vi "ReadINIfile.vi"(6 "Delete INI File First? (F)":bool, 8 "error in (no error)":errorcluster) -> (0 "error out":errorcluster, 2 "Existing Addresses":string[][](array[string]), 3 "refnum out":T1)   [LabVIEW 2009]
uses:
  <vilib>/Utility/config.llb/Config Data RefNum.ctl
  <vilib>/Utility/config.llb/Read Key (String).vi
  <vilib>/Utility/config.llb/NI_LVConfig.lvlib
  <vilib>/Utility/config.llb/Write Key (String).vi
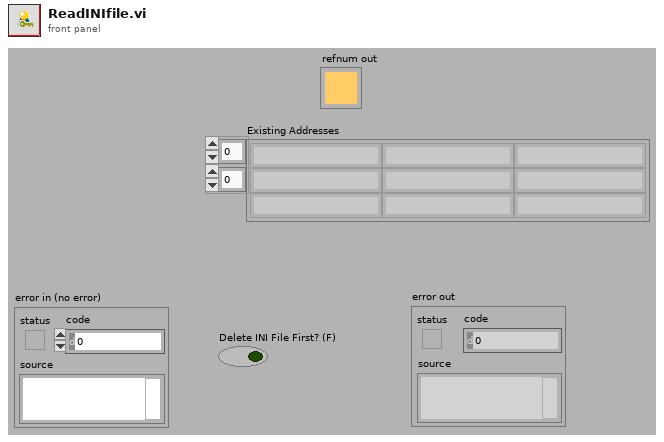
[diagram p1: front panel]
types:
  T1 = typedef "NI_LVConfig.lvlib/Config Data RefNum.ctl" = refnum<k1>
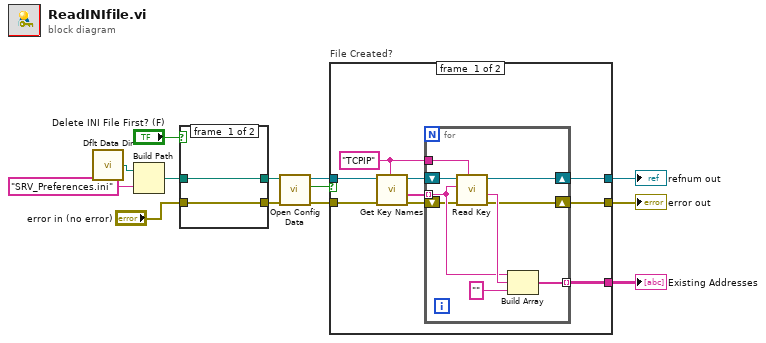
[diagram p0: block diagram]
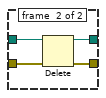
[diagram p2: hidden frame]
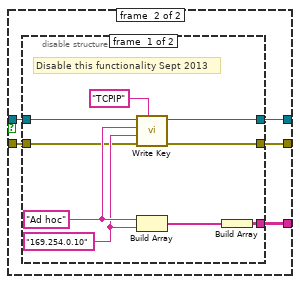
[diagram p3: hidden frame]
diagram:
  n1 = call <vilib>:"Dflt Data Dir.vi"() -> ("App:Default Data Directory"=w8:path)
  n2 = Build Path(base path=w8, name or relative path="SRV_Preferences.ini") -> (appended path=w3:path)
  n3 = case shown="True" "Delete INI File First? (F)" {
    tunnel: "error in (no error)" -> [w14 w19]
    tunnel: [w14 w18] -> w4
    tunnel: w3 -> [w15 w17]
    tunnel: [w15 w16] -> w2
    frame #0 {
    }
    frame #1 {
      n4 = Delete(path (use dialog)=w17, error in=w19) -> (deleted path=w16:path, error out=w18:errorcluster)  [unwired: 3 in, 1 out]
    }
  }
  n5 = call <vilib>:"Open Config Data.vi"("error in (no error)"=w4, "configuration file path"=w2) -> ("error out"=w7:errorcluster, "file created?"=w13:bool, "refnum"=w10:T1)  [unwired: 7 in]
  n6 = case "File Created?" shown="True" w13 {
    tunnel: w10 -> [w28 w42]
    tunnel: [w21 w41] -> w11
    tunnel: [w25 w40] -> w12
    tunnel: w7 -> [w24 w39]
    tunnel: [w20 w38] -> w6
    frame #0 {
      w27 = "TCPIP" ("section")
      n7 = call <vilib>:"Get Key Names.vi"("section"=w27, "error in (no error)"=w24, "refnum"=w28) -> ("error out"=w23:errorcluster, "key names"=w26:string[], "refnum out"=w22:T1)  [unwired: 5 in, 1 out]
      n8 = for {
        tunnel: w27 -> [w36]
        tunnel: w26 -> [w32] mode=indexing
        tunnel: [w34] -> w25 mode=indexing
        shift-right: [w30] -> w20
        shift-left: w23 -> [w31]
        shift-right: [w29] -> w21
        shift-left: w22 -> [w37]
        n9 = call-poly <vilib>:"Read Key.vi"("section"=w36, "error in (no error)"=w31, "key"=w32, "refnum"=w37) -> ("error out"=w30:errorcluster, "value"=w35:string, "refnum out"=w29:T1)  [unwired: 4 in, 1 out]
        n10 = Build Array(w32, w35, "" ("section")) -> (w34:string[])
      }
    }
    frame #1 {
      n11 = disable-structure shown="Enabled" {
        disable-tunnel: w42 -> [w50 w53]
        disable-tunnel: [w49 w53] -> w41
        disable-tunnel: [w45 _] -> w40
        disable-tunnel: w39 -> [w44 w52]
        disable-tunnel: [w43 w52] -> w38
        frame #0 {
          w48 = "Ad hoc" ("key")
          w47 = "169.254.0.10" ("key")
          # "Disable this functionality Sept 2013"
          n12 = call-poly <vilib>:"Write Key.vi"("section"="TCPIP", "error in (no error)"=w44, "value"=w47, "key"=w48, "refnum"=w50) -> ("error out"=w43:errorcluster, "refnum out"=w49:T1)  [unwired: 4 in, 1 out]
          n13 = Build Array(w48, w47) -> (w46:string[])
          n14 = Build Array(w46) -> (w45:string[][])
        }
        frame #1 {
        }
      }
    }
  }
  "Existing Addresses" <- w12
  "refnum out" <- w11
  "error out" <- w6
